vi "WSVCAP SHL FPGA LL RFFE Debug Global.vi"() -> ()   [LabVIEW 2012]
panel:
  out "Sim Write Memory":u16[](array[numeric]) format="%08x"
  in  "RFFE CH (1-16)":i32
  in  "RFFE_DATO":bool
  in  "RFFE_DAA":bool
  in  "RFFE_CLK":bool
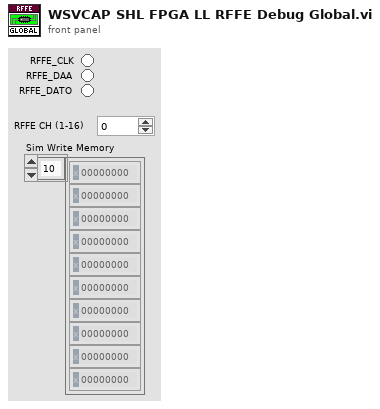
[diagram p1: front panel]
diagram:
